vi "Load and Save Data (IQ Data).vi"(0 "VISA resource name":refnum<visa-resource-name>, 1 "I/Q Symbols Values":cdb[](array[numeric])=[0.0+0.0i, 0.0+0.0i], 2 "Differential States Count (2)":u32=2, 5 "Destination File":string, 7 "Enable Q Output Delay(T:Enable)":bool=TRUE, 9 "Symbols Count (2)":u32=2, 11 "error in (no error)":errorcluster, 12 "Enable Differential Encoding (F:Disable)":bool, 13 "Differential States":dbl[](array[numeric])=[0.0, 0.0]) -> (4 "VISA resource name out":refnum<visa-resource-name>, 15 "error out":errorcluster)   [LabVIEW 2018, in "Agilent PSG MXG Series.lvlib"]
doc: "Loads custom I/Q data into a file in the signal generator's non-volatile memory.\n\n<B>Notes:</B>\n(1) This VI is valid in N5172B that installs with <B>Option 653</B> or <B>Option 655</B>, or N5182B that installs with <B>Option 656</B> or <B>Option 657</B>.\n(2) This VI is valid in N5162A/82A that installs with <B>Option 651</B>, <B>Option 652</B>, or <B>Option 654</B>."
uses:
  Agilent PSG MXG Series.lvlib
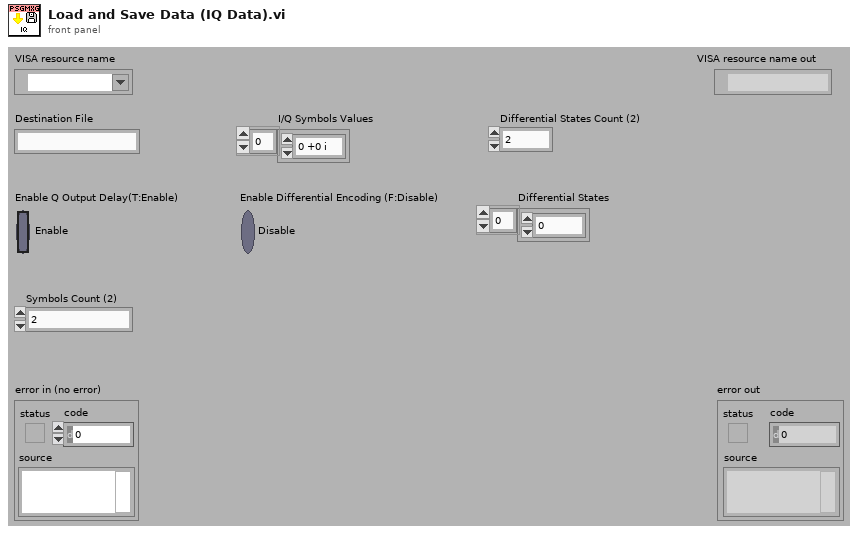
[diagram p1: front panel]
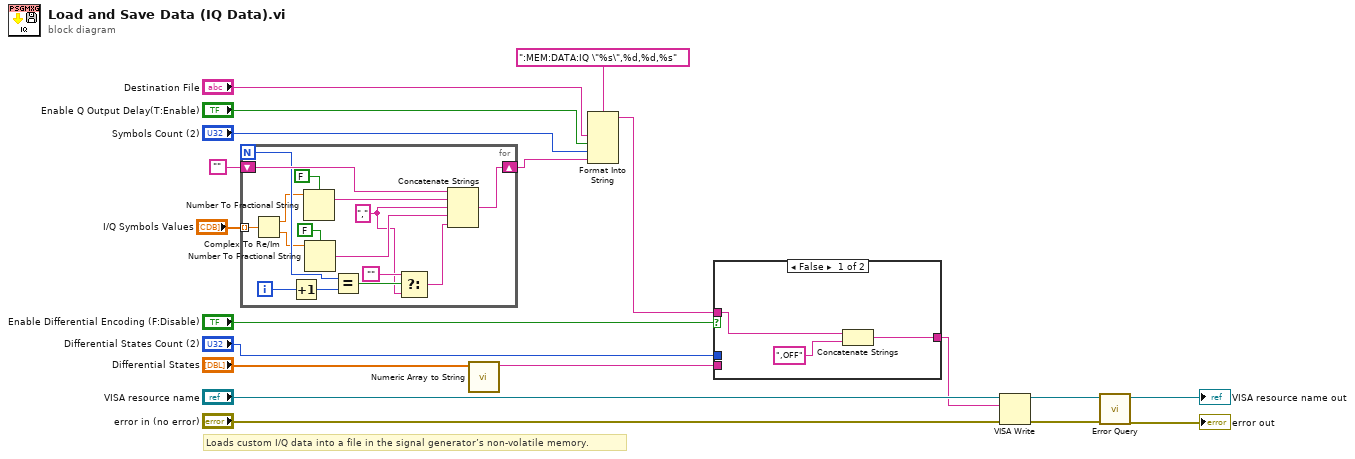
[diagram p0: block diagram]
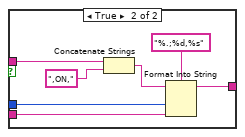
[diagram p2: hidden frame]
diagram:
  # "Loads custom I/Q data into a file in the signal generator’s non-volatile memory."
  n1 = for {
    N -> [w29]
    shift-right: [w33] -> w2
    shift-left: "" -> [w32]
    tunnel: "I/Q Symbols Values" -> [w24] mode=indexing
    i -> [w31]
    w25 = "," ("string")
    n2 = Complex To Re/Im(x + iy=w24) -> (x=w23:dbl, y=w22:dbl)
    n3 = Increment(x=w31) -> (x+1=w30:i32)
    n4 = Number To Fractional String(use system decimal point (T)=FALSE, number=w23) -> (F-format string=w35:string)  [unwired: 2 in]
    n5 = Number To Fractional String(use system decimal point (T)=FALSE, number=w22) -> (F-format string=w34:string)  [unwired: 2 in]
    n6 = Equal?(x=w29, y=w30) -> (x = y?=w28:bool)
    n7 = Select(t="", s=w28, f=w25) -> (s? t:f=w27:string)
    n8 = Concatenate Strings(w32, w35, w25, w34, w27) -> (w33:string)
  }
  n9 = call "Numeric Array to String.vi"("Numeric Array"="Differential States") -> ("Output String"=w8:string)  [unwired: 10 in]
  n10 = Format Into String(format string=":MEM:DATA:IQ \"%s\",%d,%d,%s", "Destination File", "Enable Q Output Delay(T:Enable)", "Symbols Count (2)", w2) -> (resulting string=w10:string)  [unwired: 2 in, 1 out]
  n11 = case shown="False" "Enable Differential Encoding (F:Disable)" {
    tunnel: w10 -> [w38 w44]
    tunnel: [w36 w39] -> w9
    tunnel: w8 -> [_ w40]
    tunnel: "Differential States Count (2)" -> [_ w41]
    frame False {
      n12 = Concatenate Strings(w38, ",OFF" ("f")) -> (w36:string)
    }
    frame True {
      n13 = Concatenate Strings(w44, ",ON,") -> (w43:string)
      n14 = Format Into String(format string="%.;%d,%s", initial string=w43, w41, w40) -> (resulting string=w39:string)  [unwired: 1 in, 1 out]
    }
  }
  n15 = VISA Write(VISA resource name="VISA resource name", write buffer=w9, error in (no error)="error in (no error)") -> (VISA resource name out=w19:refnum<visa-resource-name>, error out=w18:errorcluster)  [unwired: 1 out]
  n16 = call "Error Query.vi"("error in (no error)"=w18, "VISA resource name"=w19) -> ("error out"=→"error out":errorcluster, "VISA resource name out"=→"VISA resource name out":refnum<visa-resource-name>)  [unwired: 6 in, 2 out]
